vi "Release.vi"(8 "Error In":errorcluster, 11 "OPI Ref":refnum<data-value>) -> (0 "Error Out":errorcluster)   [LabVIEW 2012, in "OPI.lvclass"]
doc: "Stop the PES OPI Client handler and release all local data used for communication. \n\nIf this was the last connection to the PES, it will also stop."
uses:
  OPI.lvclass
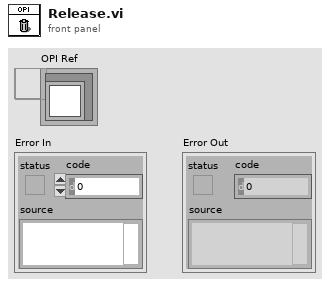
[diagram p1: front panel]
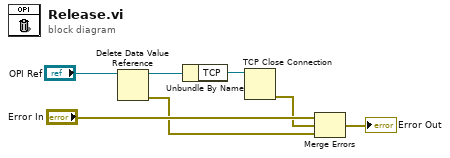
[diagram p0: block diagram]
diagram:
  n1 = Delete Data Value Reference(data value reference="OPI Ref") -> (data value=w6:refnum<class "OPI.lvclass">, error out=w2:errorcluster)  [unwired: 1 in]
  n2 = Unbundle By Name(w6) -> ("TCP"=w5:refnum<k5>)
  n3 = TCP Close Connection(connection ID=w5) -> (error out=w3:errorcluster)  [unwired: 2 in, 1 out]
  n4 = Merge Errors("Error In", w3, w2) -> (→"Error Out":errorcluster)
